vi "new failure.vi"() -> (1 "failure":T1 {"code" format="%.0x"})   [LabVIEW 2013, in "failure.lvlib"]
uses:
  failure.lvlib
  failure.ctl
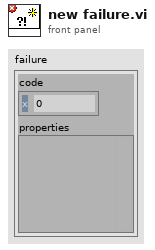
[diagram p1: front panel]
types:
  T1 = typedef "failure.lvlib/failure.ctl" = cluster{"code":i32, "properties":variant}
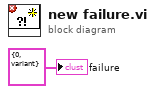
[diagram p0: block diagram]
diagram:
  "failure" <- T1 {"code"=0, "properties"=variant} ("failure")
